vi "Configure NF Monitor Spectrum Frequency.vi"(0 "VISA resource name":refnum<visa-resource-name>, 5 "Center Frequency (1.5 GHz)":dbl=1500000000.0 format="%^#_6g", 7 "Frequency Span (2.99 GHz)":dbl=2990000000.0 format="%^#_6g", 11 "error in (no error)":errorcluster, 12 "Auto Frequency Offset (Enabled)":bool=TRUE, 13 "Manual Frequency Offset (0 Hz)":dbl format="%^#_6g") -> (4 "VISA resource name out":refnum<visa-resource-name>, 15 "error out":errorcluster)   [LabVIEW 2014, in "Agilent ESA PSA Series.lvlib"]
doc: "Configures the frequency settings of the Monitor Spectrum measurement of the Noise Figure personality.\n\n<B>Note:</B> \n\nThis VI is only valid in Noise Figure personality. Use <B>Switch Personality</B> VI to switch to Noise Figure before calling this VI."
uses:
  Agilent ESA PSA Series.lvlib
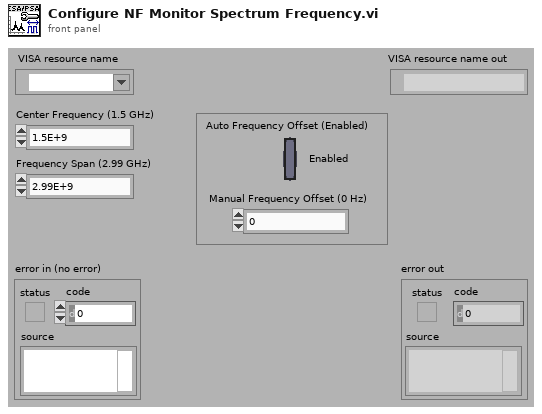
[diagram p1: front panel]
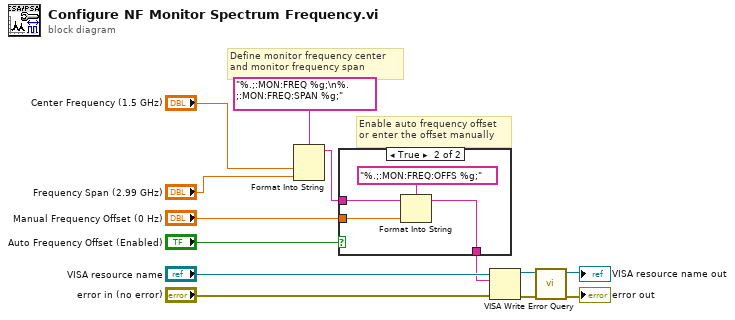
[diagram p0: block diagram]
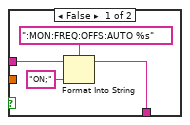
[diagram p2: hidden frame]
diagram:
  # "Enable auto frequency offset\nor enter the offset manually"
  # "Define monitor frequency center\nand monitor frequency span"
  n1 = Format Into String(format string="%.;:MON:FREQ %g;\n%.;:MON:FREQ:SPAN %g;", "Center Frequency (1.5 GHz)", "Frequency Span (2.99 GHz)") -> (resulting string=w5:string)  [unwired: 2 in, 1 out]
  n2 = case shown="True" "Auto Frequency Offset (Enabled)" {
    tunnel: w5 -> [w16 w20]
    tunnel: "Manual Frequency Offset (0 Hz)" -> [_ w21]
    tunnel: [w17 w18] -> w3
    frame False {
      n3 = Format Into String(format string=":MON:FREQ:OFFS:AUTO %s", initial string=w16, "ON;" ("input 1")) -> (resulting string=w17:string)  [unwired: 1 in, 1 out]
    }
    frame True {
      n4 = Format Into String(format string="%.;:MON:FREQ:OFFS %g;", initial string=w20, w21) -> (resulting string=w18:string)  [unwired: 1 in, 1 out]
    }
  }
  n5 = VISA Write(VISA resource name="VISA resource name", write buffer=w3, error in (no error)="error in (no error)") -> (VISA resource name out=w11:refnum<visa-resource-name>, error out=w10:errorcluster)  [unwired: 1 out]
  n6 = call "Error Query.vi"("error in (no error)"=w10, "VISA resource name"=w11) -> ("error out"=→"error out":errorcluster, "VISA resource name out"=→"VISA resource name out":refnum<visa-resource-name>)  [unwired: 6 in, 2 out]
